vi "LogHexapodData.vi"(0 "LogFilePath":path, 5 "TimeStampTreshold":dbl format="%<%H:%M:%S%1u\n%x>T", 7 "X IN":cluster{dbl[], dbl[]}[](array[cluster]) {"?" format="%<%H:%M:%S%1u\n%x>T"}, 9 "Y IN":cluster{dbl[], dbl[]}[](array[cluster]) {"?" format="%<%H:%M:%S%1u>T"}, 11 "Cumul IN":cluster{dbl[], dbl[]}[](array[cluster]) {"?" format="%<%H:%M:%S%1u>T"}) -> (15 "String":string)   [LabVIEW 2011]
panel:
  out "length":i32
  out "size_ap":i32
  out "size_av":i32
  out "TresholdIndex":i32
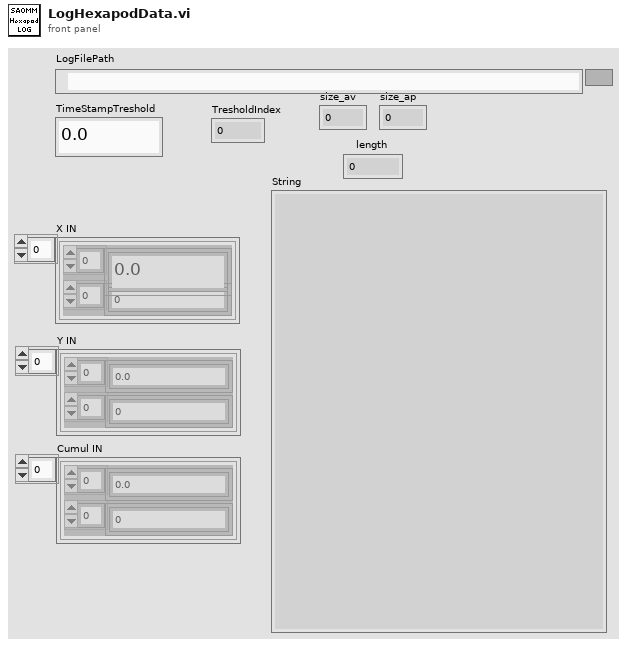
[diagram p1: front panel]
types:
  T1 = typedef "LVDateTimeRec.ctl" = cluster{"fractional second":dbl, "second":i32, "minute":i32, "hour":i32, "day of month":i32, "month":i32, "year":i32, "day of week":i32, "day of year":i32, "DST":i32}
  T2 = enum16{"open", "replace", "create", "open or create", "replace or create", "replace or create with confirmation"}
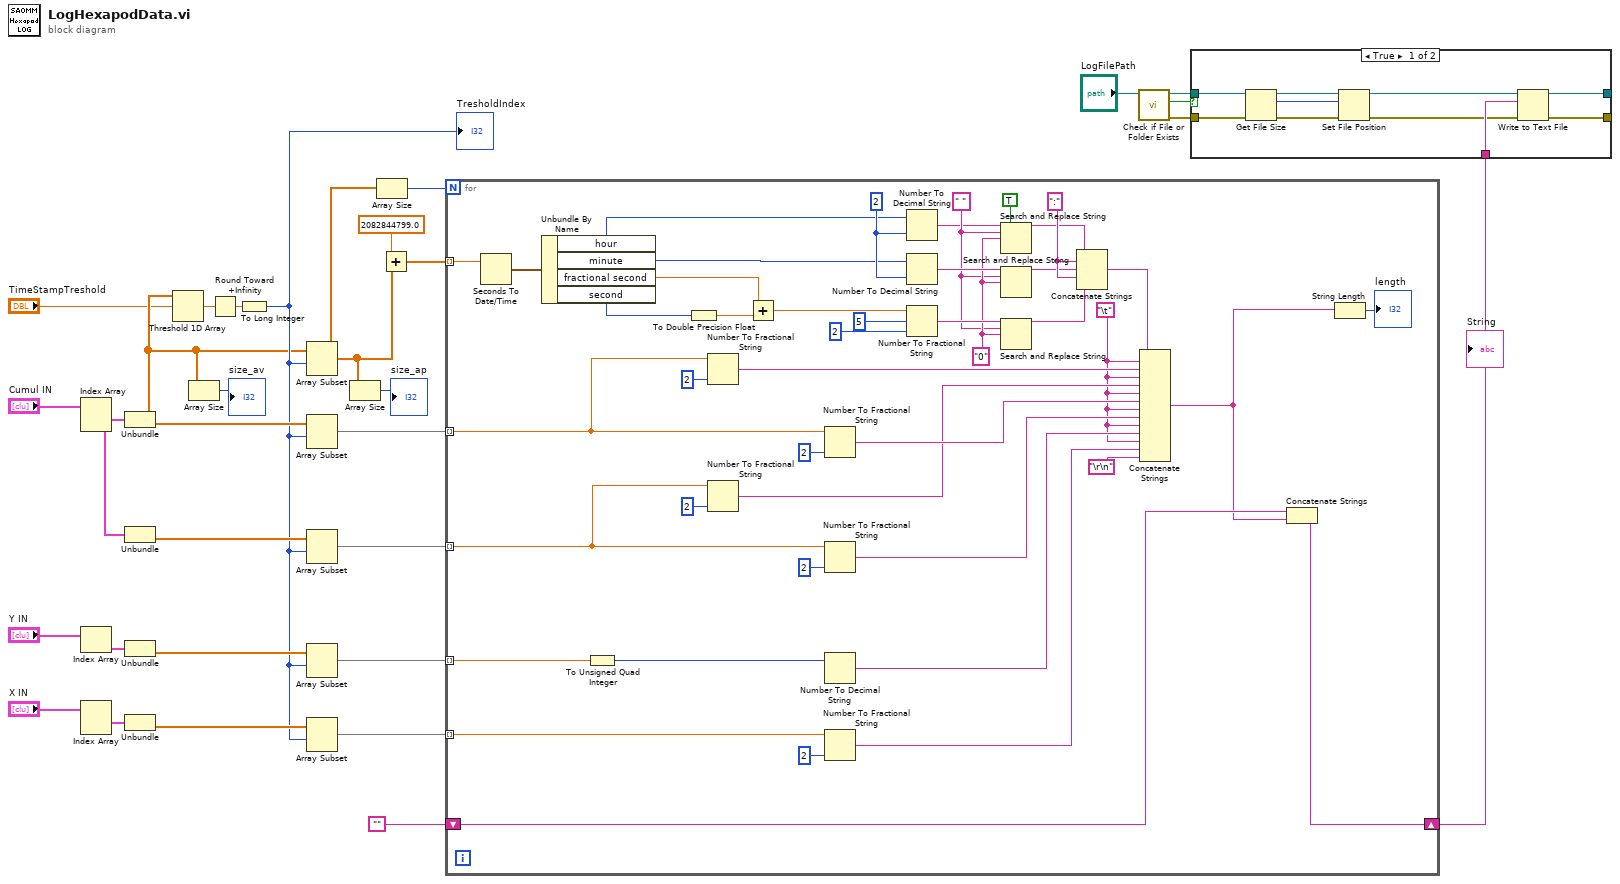
[diagram p0: block diagram]
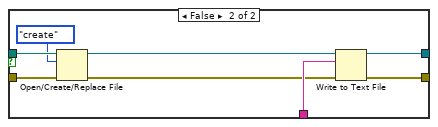
[diagram p2: hidden frame]
diagram:
  n1 = Index Array(array="Cumul IN") -> (element #1=w32:cluster{dbl[], dbl[]}, element #2=w29:cluster{dbl[], dbl[]})  [unwired: 2 in]
  n2 = Index Array(array="Y IN") -> (element=w27:cluster{dbl[], dbl[]})  [unwired: 1 in]
  n3 = Index Array(array="X IN") -> (element #1=w26:cluster{dbl[], dbl[]})  [unwired: 2 in, 1 out]
  n4 = Unbundle(w32) -> (w14:dbl[], w30:dbl[])
  n5 = Unbundle(w29) -> (w28:dbl[])  [unwired: 1 out]
  n6 = Unbundle(w27) -> (w25:dbl[])  [unwired: 1 out]
  n7 = Unbundle(w26) -> (w24:dbl[])  [unwired: 1 out]
  n8 = Threshold 1D Array(2:"TimeStampTreshold", 3:w14) -> (0:w31:dbl)  [unwired: 1 in]
  n9 = Array Size(array=w14) -> (size(s)=→"size_av":i32)
  n10 = Round Toward +Infinity(x=w31) -> (ceil(x): smallest int >= x=w23:dbl)
  n11 = To Long Integer(number=w23) -> (32bit integer=w22:i32)
  "TresholdIndex" <- w22
  n12 = Array Subset(array=w14, index=w22) -> (w3:dbl[])  [unwired: 1 in]
  n13 = Array Subset(array=w30, index=w22) -> (w10:dbl[])  [unwired: 1 in]
  n14 = Array Subset(array=w28, index=w22) -> (w11:dbl[])  [unwired: 1 in]
  n15 = Array Subset(array=w25, index=w22) -> (w20:dbl[])  [unwired: 1 in]
  n16 = Array Subset(array=w24, index=w22) -> (w19:dbl[])  [unwired: 1 in]
  n17 = Array Size(array=w3) -> (size(s)=→"size_ap":i32)
  n18 = Array Size(array=w3) -> (size(s)=w21:i32)
  n19 = Add(x=2082844799.0, y=w3) -> (x+y=w2:dbl[])
  n20 = for {
    N: w21 -> [_]
    tunnel: w2 -> [w37] mode=indexing
    tunnel: w10 -> [w40] mode=indexing
    tunnel: w11 -> [w39] mode=indexing
    tunnel: w20 -> [w56] mode=indexing
    tunnel: w19 -> [w62] mode=indexing
    shift-right: [w45] -> w5
    shift-left: "" -> [w51]
    w46 = "\t"
    w76 = ":"
    w69 = "0" ("replace string (\"\")")
    w68 = " " ("search string")
    w66 = i16 2 ("width (-)")
    n21 = Seconds To Date/Time(time stamp (now)=w37) -> (date time rec=w38:T1)  [unwired: 1 in]
    n22 = Unbundle By Name(w38) -> ("hour"=w65:i32, "minute"=w64:i32, "fractional second"=w34:dbl, "second"=w36:i32)
    n23 = To Unsigned Quad Integer(1:w56) -> (0:w55:u64)
    n24 = To Double Precision Float(number=w36) -> (double precision float=w35:dbl)
    n25 = Number To Fractional String(number=w40, precision (6)=i16 2) -> (F-format string=w47:string)  [unwired: 2 in]
    n26 = Number To Fractional String(number=w39, precision (6)=i16 2) -> (F-format string=w48:string)  [unwired: 2 in]
    n27 = Add(x=w34, y=w35) -> (x+y=w33:dbl)
    n28 = Number To Fractional String(number=w40, precision (6)=i16 2) -> (F-format string=w58:string)  [unwired: 2 in]
    n29 = Number To Fractional String(number=w39, precision (6)=i16 2) -> (F-format string=w57:string)  [unwired: 2 in]
    n30 = Number To Decimal String(number=w55) -> (decimal integer string=w54:string)  [unwired: 1 in]
    n31 = Number To Fractional String(number=w62, precision (6)=i16 2) -> (F-format string=w53:string)  [unwired: 2 in]
    n32 = Number To Decimal String(number=w65, width (-)=w66) -> (decimal integer string=w67:string)
    n33 = Number To Decimal String(number=w64, width (-)=w66) -> (decimal integer string=w70:string)
    n34 = Number To Fractional String(number=w33, width (-)=i16 5, precision (6)=i16 2) -> (F-format string=w71:string)  [unwired: 1 in]
    n35 = Search and Replace String(replace all?=TRUE ("replace all? (F)"), input string=w67, search string=w68, replace string=w69) -> (result string=w74:string)  [unwired: 4 in, 3 out]
    n36 = Search and Replace String(input string=w70, search string=w68, replace string=w69) -> (result string=w73:string)  [unwired: 5 in, 3 out]
    n37 = Search and Replace String(input string=w71, search string=w68, replace string=w69) -> (result string=w75:string)  [unwired: 5 in, 3 out]
    n38 = Concatenate Strings(w74, w76, w73, w76, w75) -> (w63:string)
    n39 = Concatenate Strings(w63, w46, w47, w46, w48, w46, w58, w46, w57, w46, w54, w46, w53, "\r\n") -> (w43:string)
    n40 = Concatenate Strings(w51, w43) -> (w45:string)
    n41 = String Length(string=w43) -> (length=→"length":i32)
  }
  "String" <- w5
  n42 = call <vilib>:"Check if File or Folder Exists.vi"("path"="LogFilePath") -> ("error out"=w6:errorcluster, "file or folder exists?"=w8:bool, "dup path"=w7:path)  [unwired: 8 in]
  n43 = case shown="True" w8 {
    tunnel: w7 -> [w80 w94]
    tunnel: w6 -> [w79 w93]
    tunnel: [w86 w92] -> _
    tunnel: [w85 w91] -> _
    tunnel: w5 -> [w84 w90]
    frame True {
      n44 = Get File Size(file=w80, error in=w79) -> (refnum out=w83:refnum<file>, size (in bytes)=w82:i64, 0:w81:errorcluster)
      n45 = Set File Position(offset (in bytes) (0)=w82, refnum=w83, error in=w81) -> (refnum out=w78:refnum<file>, error out=w77:errorcluster)  [unwired: 1 in]
      n46 = Write to Text File(file (use dialog)=w78, text=w84, error in=w77) -> (refnum out=w86:refnum<file>, error out=w85:errorcluster)  [unwired: 1 in, 1 out]
    }
    frame False {
      n47 = Open/Create/Replace File(file path (use dialog)=w94, error in=w93, operation (0:open)=T2."create") -> (refnum out=w88:refnum<file>, error out=w87:errorcluster)  [unwired: 3 in, 1 out]
      n48 = Write to Text File(file (use dialog)=w88, text=w90, error in=w87) -> (refnum out=w92:refnum<file>, error out=w91:errorcluster)  [unwired: 1 in, 1 out]
    }
  }
